vi "fpga.sandbox.vi"(0 "ip.reset":bool, 1 "TDATA":u64, 2 "TKEEP":u8, 3 "TVALID":bool, 4 "TLAST":bool, 5 "TUSER":bool) -> ()   [LabVIEW 2025]
uses:
  <vilib>/rvi/Emulation/niFpgaEmulationIsFPGAContextNoSignature.vi
  <vilib>/rvi/Emulation/niFpgaSctlEmulationGetInTimedLoop.vi
  <vilib>/rvi/errors/niFpgaSetErrorForExecOnDevCompSimple.vi
  <vilib>/rvi/eio/common/nirviEmuReportErrorAndStop.vi
  <vilib>/rvi/DataTransferAndStorage/Container/Common/niFpgaContainerGetUniqueNameForEmu.vi
  <vilib>/rvi/FIFO/Fifo_Resource/nirvififoEmulationSetSize.vi
  <vilib>/rvi/FIFO/Fifo_Resource/nirviFifoEmulationQueueMgr.vi
  <instcachedir>/0/nirviFifoEmulationQueueMgr_E5CAEC123FF24DC58D834DCA3CDAA9B5.lvgen/nirviFifoEmulationQueueMgr_E5CAEC123FF24DC58D834DCA3CDAA9B5_002.vi
  <vilib>/rvi/FIFO/Fifo_Resource/nirvififoEmulationDetermineInputValidOut.vi
  <vilib>/rvi/FIFO/Fifo_Resource/nirvififoEmulationCreateLock.vi
  <vilib>/rvi/Emulation/niFpgaProcessEmulError.vi
  <vilib>/rvi/FIFO/Fifo_Resource/nirvififoEmulationObtainLock.vi
  <vilib>/rvi/FIFO/Fifo_Resource/nirvififoEmulationReleaseLock.vi
  <vilib>/rvi/occurrence/nirviWaitOnOccurrenceBase.vi
  <vilib>/rvi/errors/nirviReportUnexpectedCaseInternalError.vi
  <vilib>/rvi/errors/nirviReportUnexpectedCaseInternalError (U32).vi
  <vilib>/rvi/DataTransferAndStorage/Container/XNode/niFpgaContainer.xnode
  <vilib>/rvi/FIFO/Fifo_Resource/nirvififoEmulationWrite.vi
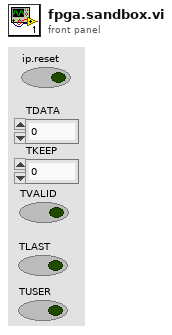
[diagram p1: front panel]
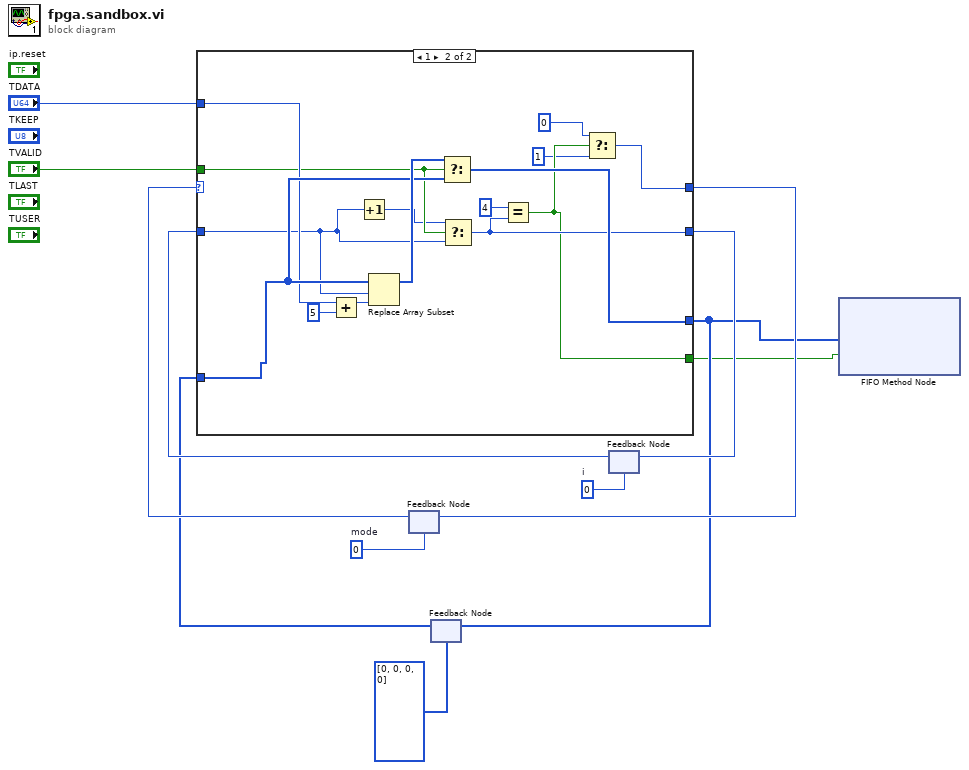
[diagram p0: block diagram]
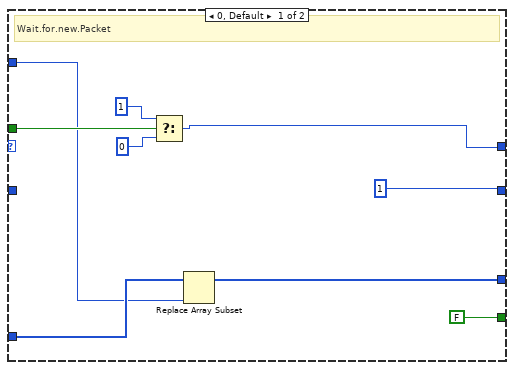
[diagram p2: hidden frame]
diagram:
  w9 = u8 0  # i
  w10 = u8 0  # mode
  n1 = feedback #1(w10) -> (w11:u8)
  n2 = feedback #2(u64[] [0, 0, 0, 0]) -> (w3:u64[])
  n3 = feedback #3(w9) -> (w8:u8)
  n4 = case shown="1" w11 {
    tunnel: [w21 w25] -> w12
    tunnel: w8 -> [_ w31]
    tunnel: [u8 1 ("f") w29] -> w7
    tunnel: "TVALID" -> [w18 w32]
    tunnel: "TDATA" -> [w15 w33]
    tunnel: w3 -> [w16 w35]
    tunnel: [w14 w34] -> w2
    tunnel: [FALSE w27] -> w1
    frame 0, Default {
      # "Wait.for.new.Packet"
      n5 = Select(t=u8 1, s=w18, f=u8 0) -> (s? t:f=w21:u8)
      n6 = Replace Array Subset(array=w16, new element=w15) -> (w14:u64[])  [unwired: 1 in]
    }
    frame 1 {
      n7 = Add(x=w33, y=u64 5) -> (x+y=w23:u64)
      n8 = Increment(x=w31) -> (x+1=w30:u8)
      n9 = Replace Array Subset(array=w35, new element=w23, index=w31) -> (w36:u64[])
      n10 = Select(t=w36, s=w32, f=w35) -> (s? t:f=w34:u64[])
      n11 = Select(t=w30, s=w32, f=w31) -> (s? t:f=w29:u8)
      n12 = Equal?(x=u8 4, y=w29) -> (x = y?=w27:bool)
      n13 = Select(t=u8 0, s=w27, f=u8 1 ("t")) -> (s? t:f=w25:u8)
    }
  }
  n14 = feedback-in #1(w12) -> ()
  n15 = feedback-in #2(w2) -> ()
  n16 = feedback-in #3(w7) -> ()
  n17 = xnode ("FIFO Method Node")("Element"=w2, "Input Valid"=w1) -> ()  [unwired: 1 in, 2 out]
